vi "入队.vi"(9 "输入点":cluster{"x":dbl, "y":dbl}, 10 "数组输入":cluster{"x":dbl, "y":dbl}[](array[cluster]), 11 "地图":u32[][](array[colorbox])) -> (2 "数组输出":cluster{"x":dbl, "y":dbl}[](array[cluster]), 3 "地图 2":u32[][](array[colorbox]))   [LabVIEW 2012]
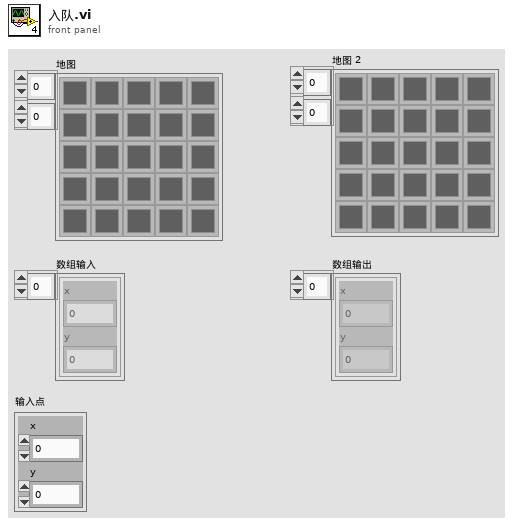
[diagram p1: front panel]
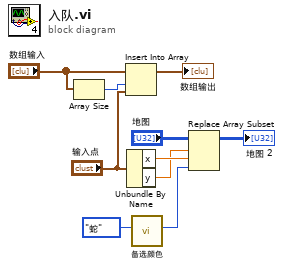
[diagram p0: block diagram]
diagram:
  n1 = Array Size(array="数组输入") -> (size(s)=w9:i32)
  n2 = Insert Into Array(array="数组输入", index=w9, new element="输入点") -> (→"数组输出":cluster{"x":dbl, "y":dbl}[])
  n3 = Unbundle By Name("输入点") -> ("x"=w5:dbl, "y"=w4:dbl)
  n4 = call "备选颜色.vi"("索引2"=enum16{"空白", "蛇", "食物", "墙", "传送门"}."蛇") -> ("颜色2"=w2:u32)  [unwired: 9 in, 1 out]
  n5 = Replace Array Subset(array="地图", new element=w2, index (row)=w4, index (col)=w5) -> (→"地图 2":u32[][])
